vi "galvo_functional_global.vi"(6 "Est Sweep Speed":i32=28000, 7 "State":T3=enum."Shutdown", 8 "error in (no error)":errorcluster, 9 "Trigger Source":tag="/Dev2/PFI7", 10 "Analog Output":tag="Dev2/ao0:1", 11 "user event out":refnum<user-event>) -> (0 "error out":errorcluster, 3 "Scanning Output":T1={"Fast Axis Offset"=10.0, "Slow Axis Offset"=0.0, "Slow Axis Amp"=20.0, "Fast Axis Amp"=20.0, "Scan Pattern"=enum."Raster"} {"Fast Axis Amp" max=20 format="%#.2f"; "Slow Axis Amp" max=20 format="%#.2f"; "Slow Axis Offset" max=10 format="%#.2f"; "Fast Axis Offset" max=10 format="%#.2f"})   [LabVIEW 2014]
doc: "Allows for the control of Galvos. The Initialize State requires that Channels and Trigger Source be set. The Run Raster state requires there to be scan parameters input so the proper scan pattern can be created and automatically loaded onto the card. The other states don't require an input.\n\n***Run Circle is incomplete at this time***"
uses:
  <vilib>/DAQmx/configure/timing.llb/DAQmx Timing (Sample Clock).vi
  <vilib>/DAQmx/create/channels.llb/DAQmx Create Channel (AO-Voltage-Basic).vi
  <resource>/objmgr/daqmx.rc
  <vilib>/DAQmx/write.llb/DAQmx Write (Analog 2D DBL NChan NSamp).vi
  galvo_states.ctl
  Classes/Galvo/Scanning Cluster.ctl
  Classes/Galvo/Galvo.lvclass
panel:
  in  "Scanning":T2={"Fast Axis Offset"=0.0, "Slow Axis Offset"=0.0, "Slow Axis Amp"=5.0, "Fast Axis Amp"=5.0, "Slow Axis Samples"=1, "Fast Axis Samples"=500, "Scan Pattern"=enum."Raster"} {"Fast Axis Samples" max=1000 step=1; "Slow Axis Samples" max=1000 step=1; "Fast Axis Amp" max=20 format="%#.2f"; "Slow Axis Amp" max=20 format="%#.2f"; "Slow Axis Offset" max=10 format="%#.2f"; "Fast Axis Offset" max=10 format="%#.2f"}
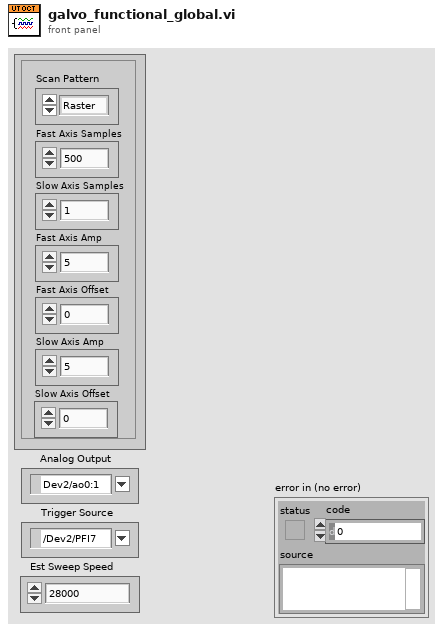
[diagram p1: front panel]
types:
  T1 = typedef "Galvo.lvclass/Scanning Cluster.ctl" = cluster{"Fast Axis Offset":sgl, "Slow Axis Offset":sgl, "Slow Axis Amp":sgl, "Fast Axis Amp":sgl, "Scan Pattern":enum16{"Raster"}}
  T2 = typedef "Galvo.lvclass/Scanning Cluster.ctl" = cluster{"Fast Axis Offset":sgl, "Slow Axis Offset":sgl, "Slow Axis Amp":sgl, "Fast Axis Amp":sgl, "Slow Axis Samples":u32, "Fast Axis Samples":u32, "Scan Pattern":enum16{"Raster"}}
  T3 = typedef "galvo_states.ctl" = enum16{"Reset", "Reset Galvos?", "Center Galvos", "Register Callback", "Get Scan Parameters", "Show", "Initialize", "Run Raster", "Load Raster", "Run Circle", "Shutdown"}
  T4 = enum32{"Invalid", "Standard", "Closed", "Hidden", "Minimized", "Maximized"}
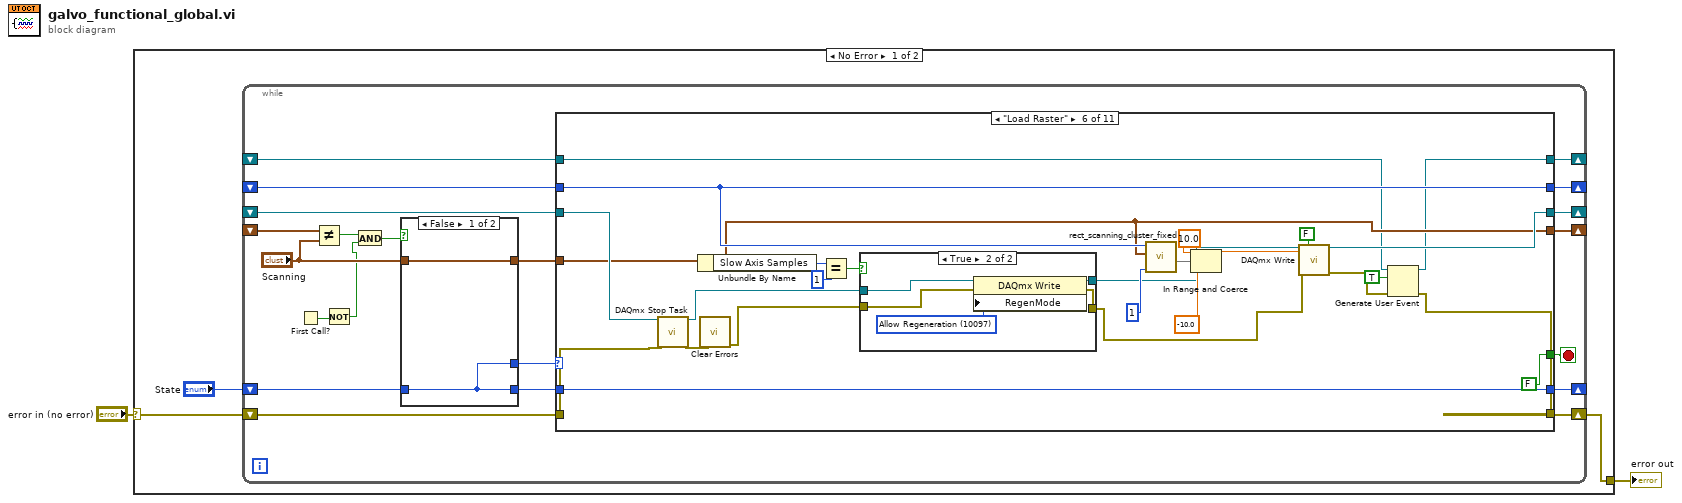
[diagram p0: block diagram]
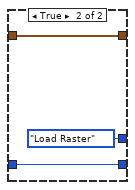
[diagram p2: hidden frame]
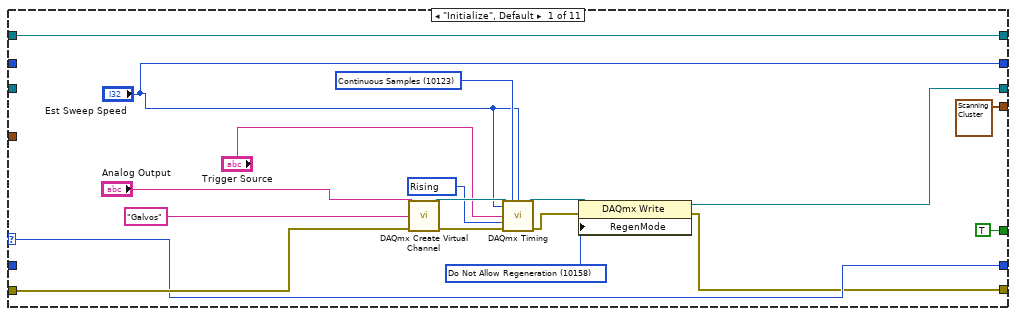
[diagram p3: hidden frame]
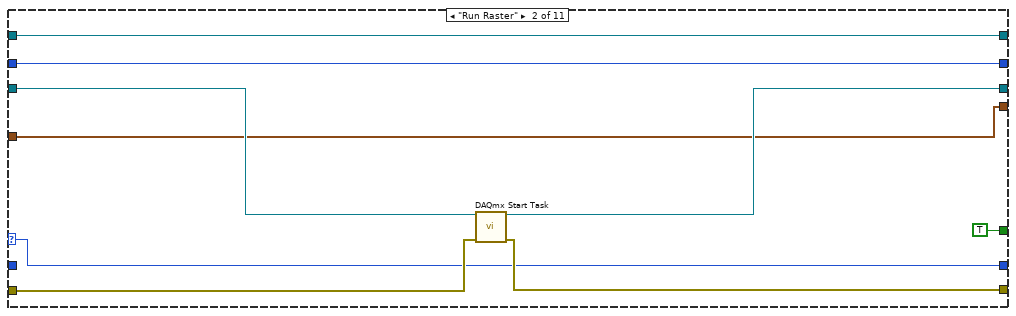
[diagram p4: hidden frame]
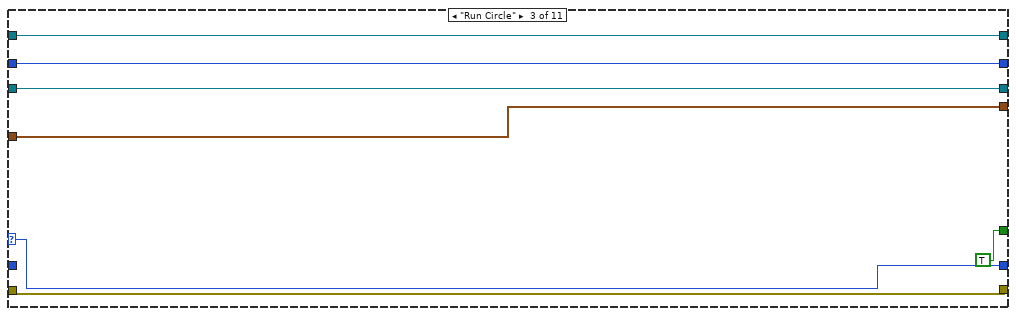
[diagram p5: hidden frame]
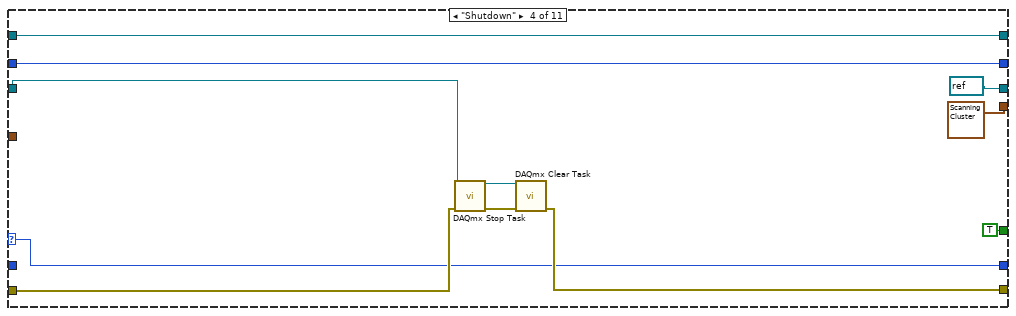
[diagram p6: hidden frame]
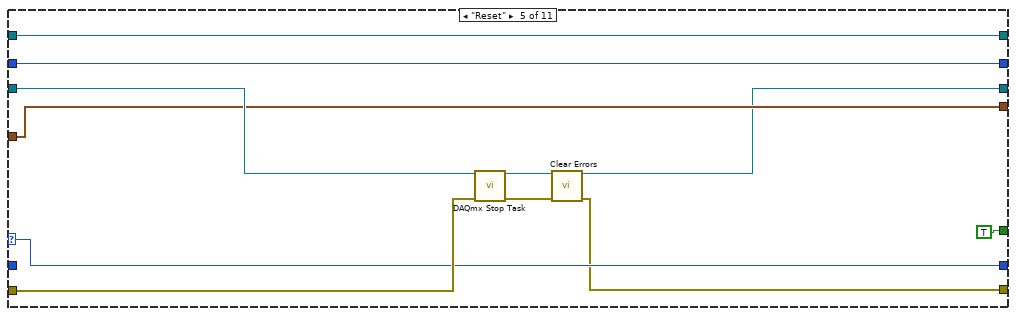
[diagram p7: hidden frame]
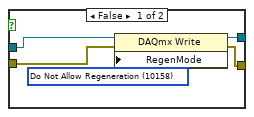
[diagram p8: hidden frame]
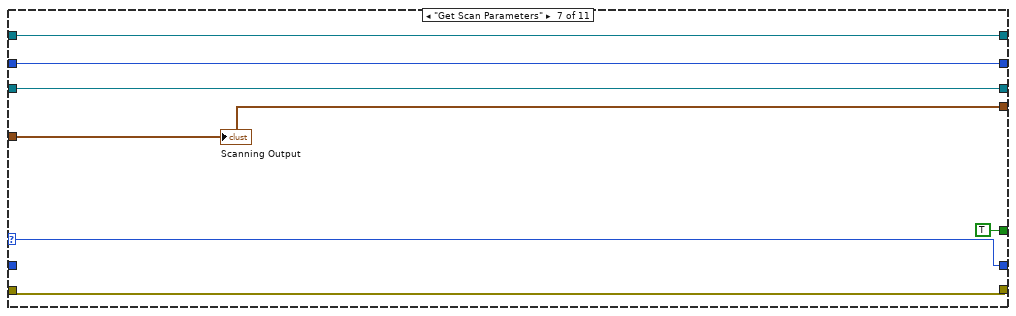
[diagram p9: hidden frame]
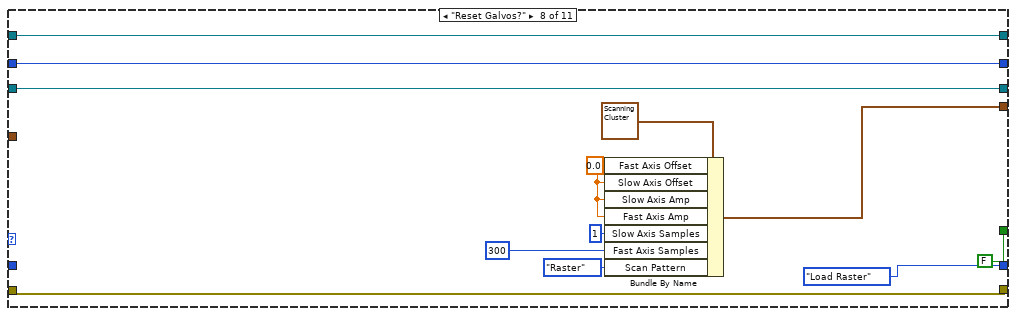
[diagram p10: hidden frame]
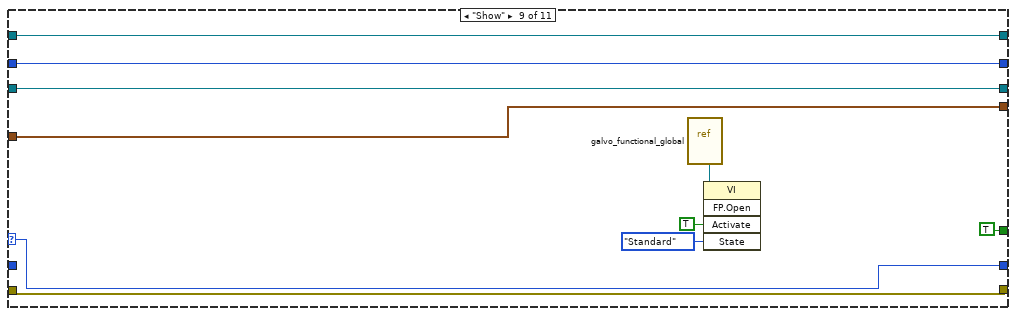
[diagram p11: hidden frame]
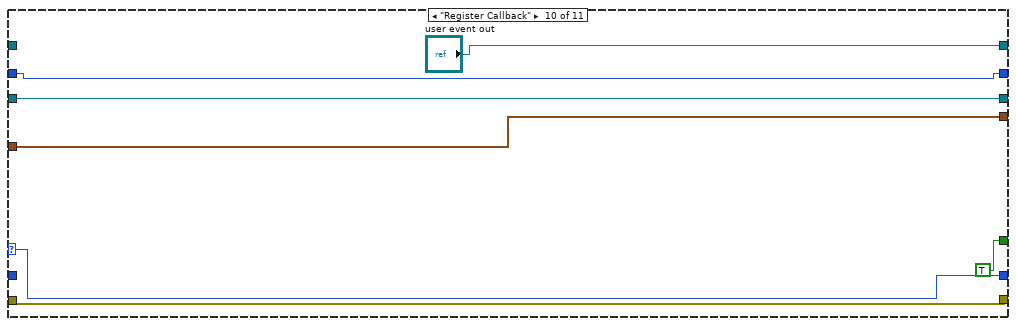
[diagram p12: hidden frame]
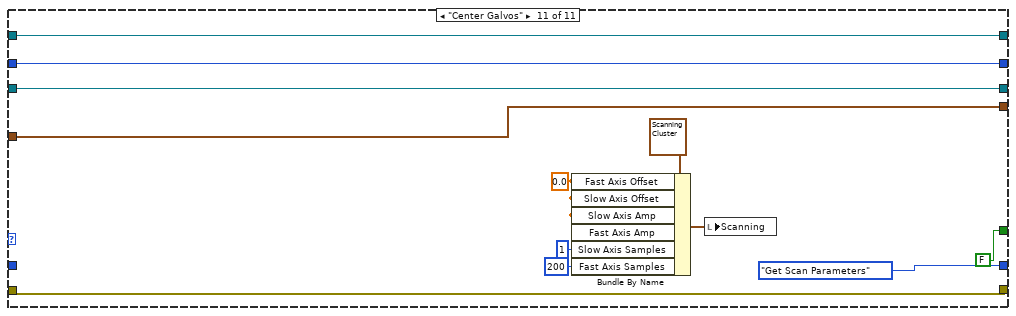
[diagram p13: hidden frame]
diagram:
  n1 = case shown="No Error" "error in (no error)" {
    selector: "error in (no error)" -> [w5 w171]
    tunnel: [w4 w171] -> w1
    frame No Error {
      n2 = while {
        shift-right: [w25] -> _
        shift-left: _ -> [w24]
        shift-right: [w23] -> w4
        shift-left: w5 -> [w26]
        shift-right: [w22] -> _
        shift-left: _ -> [w21]
        shift-right: [w20] -> _
        shift-left: _ -> [w16]
        shift-right: [w18] -> _
        shift-left: "State" -> [w15]
        shift-right: [w17] -> _
        shift-left: _ -> [w6]
        stop <- w19 stop-if-true
        n3 = First Call?() -> (First Call?: T/F=w10:bool)
        n4 = Not Equal?(x=w16, y="Scanning") -> (x != y?=w8:bool)
        n5 = Not(x=w10) -> (.not. x?=w7:bool)
        n6 = And(x=w8, y=w7) -> (x .and. y?=w9:bool)
        n7 = case shown="False" w9 {
          tunnel: w15 -> [w28 w30]
          tunnel: [w28 galvo_states."Load Raster" ("State")] -> w14
          tunnel: [w28 w30] -> w13
          tunnel: [w27 w29] -> w12
          tunnel: "Scanning" -> [w27 w29]
          frame False {
          }
          frame True {
          }
        }
        n8 = case shown="\"Load Raster\"" w14 {
          selector: w14 -> [w37 w51 w61 w68 w81 _ w123 _ w144 w153 _]
          tunnel: w26 -> [w46 w57 w64 w73 w86 w108 w127 w139 w148 w154 w160]
          tunnel: [w43 w55 w65 refnum<k21> refnum ("task out") w77 w109 w128 w140 w146 w156 w170] -> w25
          tunnel: w24 -> [_ w58 w65 w76 w85 w112 w128 w140 w146 w156 w170]
          tunnel: [w32 w56 w64 w72 w79 w110 w127 w139 w148 w154 w160] -> w23
          tunnel: ["Est Sweep Speed" w54 w63 w70 w84 w111 w129 w141 w145 w157 w169] -> w22
          tunnel: w21 -> [_ w54 w63 w70 w84 w111 w129 w141 w145 w157 w169]
          tunnel: w12 -> [_ w53 w62 _ w83 w89 w126 _ w147 w155 w162]
          tunnel: [T1 {"Fast Axis Offset"=10.0, "Slow Axis Offset"=0.0, "Slow Axis Amp"=20.0, "Fast Axis Amp"=20.0, "Scan Pattern"=enum."Raster"} ("Scanning") w53 w62 T1 {"Fast Axis Offset"=10.0, "Slow Axis Offset"=0.0, "Slow Axis Amp"=20.0, "Fast Axis Amp"=20.0, "Scan Pattern"=enum."Raster"} ("Scanning") w83 w89 w126 w130 w147 w155 w162] -> w20
          tunnel: [TRUE TRUE TRUE TRUE TRUE FALSE TRUE FALSE TRUE TRUE FALSE] -> w19
          tunnel: [w37 w51 w61 w68 w81 w90 w123 galvo_states."Load Raster" ("State") w144 w153 galvo_states."Get Scan Parameters" ("State")] -> w18
          tunnel: [w35 w50 w59 w67 w80 w87 w124 w136 w142 "user event out" w168] -> w17
          tunnel: w6 -> [w35 w50 w59 w67 w80 w88 w124 w136 w142 _ w168]
          tunnel: w13 -> [_ _ _ _ _ w90 _ _ _ _ _]
          frame "Initialize", Default {
            w42 = 10158 items=["Allow Regeneration"=10097, "Do Not Allow Regeneration"=10158] ("RegenMode")
            w47 = 10280 items=["Rising"=10280, "Falling"=10171] ("active edge")
            w45 = 10123 items=["Finite Samples"=10178, "Continuous Samples"=10123, "Hardware Timed Single Point"=12522] ("sample mode")
            n9 = call-poly <vilib>:"DAQmx Create Virtual Channel.vi"("physical channels"="Analog Output", "name to assign"="Galvos", "error in"=w46) -> ("task out"=w49:refnum<k21>, "error out"=w48:errorcluster)  [unwired: 6 in, 5 out]
            n10 = call-poly <vilib>:"DAQmx Timing.vi"("task/channels in"=w49, "sample mode"=w45, "samples per channel"="Est Sweep Speed", "rate"="Est Sweep Speed", "source"="Trigger Source", "active edge"=w47, "error in"=w48) -> ("task out"=w44:refnum<k21>, "error out"=w41:errorcluster)  [unwired: 7 out]
            n11 = property class="DAQmx Write"(reference=w44, error in=w41, "RegenMode"=w42) -> (reference out=w43:refnum<k21>, error out=w32:errorcluster)
          }
          frame "Run Raster" {
            n12 = call <vilib>:"DAQmx Start Task.vi"("task/channels in"=w58, "error in"=w57) -> ("task out"=w55:refnum<k21>, "error out"=w56:errorcluster)  [unwired: 12 in]
          }
          frame "Run Circle" {
          }
          frame "Shutdown" {
            n13 = call <vilib>:"DAQmx Stop Task.vi"("task/channels in"=w76, "error in"=w73) -> ("task out"=w75:refnum<k21>, "error out"=w74:errorcluster)  [unwired: 12 in]
            n14 = call <vilib>:"DAQmx Clear Task.vi"("task in"=w75, "error in"=w74) -> ("error out"=w72:errorcluster)  [unwired: 13 in]
          }
          frame "Reset" {
            n15 = call <vilib>:"DAQmx Stop Task.vi"("task/channels in"=w85, "error in"=w86) -> ("task out"=w77:refnum<k21>, "error out"=w78:errorcluster)  [unwired: 12 in]
            n16 = call <vilib>:"Clear Errors.vi"("error in (no error)"=w78) -> ("error out"=w79:errorcluster)  [unwired: 5 in, 1 out]
          }
          frame "Load Raster" {
            n17 = call <vilib>:"DAQmx Stop Task.vi"("task/channels in"=w112, "error in"=w108) -> ("task out"=w96:refnum<k21>, "error out"=w100:errorcluster)  [unwired: 12 in]
            n18 = Unbundle By Name(w89) -> ("Slow Axis Samples"=w99:u32)
            n19 = call <vilib>:"Clear Errors.vi"("error in (no error)"=w100) -> ("error out"=w94:errorcluster)  [unwired: 5 in, 1 out]
            n20 = Equal?(x=w99, y=u32 1) -> (x = y?=w97:bool)
            n21 = case shown="True" w97 {
              tunnel: w96 -> [w115 w121]
              tunnel: [w117 w120] -> w95
              tunnel: w94 -> [w114 w119]
              tunnel: [w113 w118] -> w93
              frame False {
                w116 = 10158 items=["Allow Regeneration"=10097, "Do Not Allow Regeneration"=10158] ("RegenMode")
                n22 = property class="DAQmx Write"(reference=w115, error in=w114, "RegenMode"=w116) -> (reference out=w117:refnum<k21>, error out=w113:errorcluster)
              }
              frame True {
                w122 = 10097 items=["Allow Regeneration"=10097, "Do Not Allow Regeneration"=10158] ("RegenMode")
                n23 = property class="DAQmx Write"(reference=w121, error in=w119, "RegenMode"=w122) -> (reference out=w120:refnum<k21>, error out=w118:errorcluster)
              }
            }
            n24 = call "rect_scanning_cluster_fixed.vi"(8:1 ("B-Scans per Buffer"), "Fast Axis"=w89, "Scanning"=w111) -> (1:w106)  [unwired: 7 in, 1 out]
            n25 = In Range and Coerce(upper limit=10.0, x=w106, lower limit=-10.0) -> (coerced(x)=w103:dbl)  [unwired: 1 out]
            n26 = call-poly <vilib>:"DAQmx Write.vi"("task/channels in"=w95, "auto start"=FALSE, "data"=w103, "error in"=w93) -> ("task out"=w109:refnum<k21>, "error out"=w92:errorcluster)  [unwired: 10 out]
            n27 = Generate User Event(user event=w88, event data cluster=TRUE ("event data"), error in=w92) -> (user event out=w87:refnum<user-event>, error out=w110:errorcluster)  [unwired: 1 in]
          }
          frame "Get Scan Parameters" {
            "Scanning Output" <- w126
          }
          frame "Reset Galvos?" {
            w134 = sgl 0.0 ("Fast Axis Offset")
            n28 = Bundle By Name(cluster=T1 {"Fast Axis Offset"=10.0, "Slow Axis Offset"=0.0, "Slow Axis Amp"=20.0, "Fast Axis Amp"=20.0, "Scan Pattern"=enum."Raster"} ("Scanning"), "Fast Axis Offset"=w134, "Slow Axis Offset"=w134, "Slow Axis Amp"=w134, "Fast Axis Amp"=w134, "Slow Axis Samples"=u32 1 ("B-scans (rings)"), "Fast Axis Samples"=u32 300 ("A(cluster)/B"), "Scan Pattern"=enum16{"Raster"}."Raster") -> (w130:T1)
          }
          frame "Show" {
            n29 = vi-ref "galvo_functional_global.vi"() -> (w151:refnum<vi>)
            n30 = invoke class="VI" method="FP.Open"(reference=w151, "Activate"=TRUE ("Activate?"), "State"=T4."Standard") -> ()  [unwired: 2 in, 5 out]
          }
          frame "Register Callback" {
          }
          frame "Center Galvos" {
            w167 = sgl 0.0 ("Fast Axis Offset")
            n31 = Bundle By Name(cluster=T2 {"Fast Axis Offset"=0.0, "Slow Axis Offset"=0.0, "Slow Axis Amp"=5.0, "Fast Axis Amp"=2.0, "Slow Axis Samples"=1, "Fast Axis Samples"=500, "Scan Pattern"=enum."Raster"} ("Scanning"), "Fast Axis Offset"=w167, "Slow Axis Offset"=w167, "Slow Axis Amp"=w167, "Fast Axis Amp"=w167, "Slow Axis Samples"=u32 1 ("B-scans (rings)"), "Fast Axis Samples"=u32 200 ("A(cluster)/B")) -> (w163:T2)
            n32 = local write "Scanning"(w163) -> ()
          }
        }
      }
    }
    frame Error {
    }
  }
  "error out" <- w1
